vi "WPI_CameraUpdate Settings.vi"(8 "Name":string, 9 "Table":string, 11 "CameraDevRef":T1) -> ()   [LabVIEW 2017]
uses:
  <vilib>/Rock Robotics/WPI/Camera/WPI_CameraDevRef.ctl
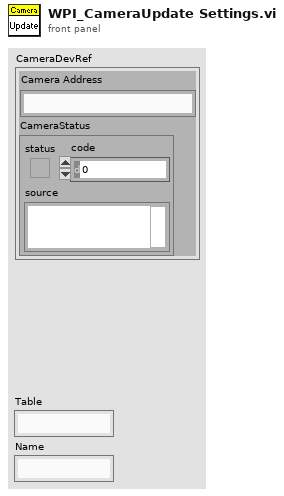
[diagram p1: front panel]
types:
  T1 = typedef "WPI_CameraDevRef.ctl" = cluster{"Camera Address":string, "CameraStatus":errorcluster}
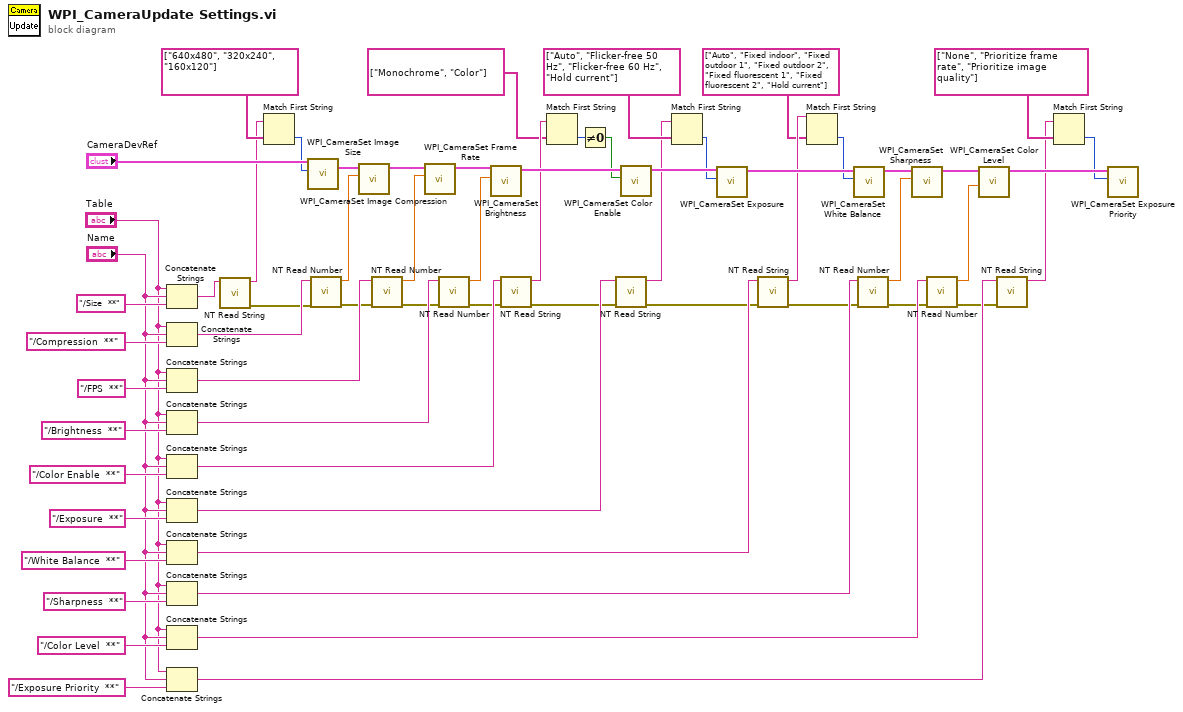
[diagram p0: block diagram]
diagram:
  n1 = Concatenate Strings("Table", "Name", "/Size  **") -> (w40:string)
  n2 = Concatenate Strings("Table", "Name", "/Compression  **") -> (w39:string)
  n3 = Concatenate Strings("Table", "Name", "/FPS  **") -> (w38:string)
  n4 = Concatenate Strings("Table", "Name", "/Brightness  **") -> (w37:string)
  n5 = Concatenate Strings("Table", "Name", "/Color Enable  **") -> (w14:string)
  n6 = Concatenate Strings("Table", "Name", "/Exposure  **") -> (w36:string)
  n7 = Concatenate Strings("Table", "Name", "/White Balance  **") -> (w35:string)
  n8 = Concatenate Strings("Table", "Name", "/Sharpness  **") -> (w34:string)
  n9 = Concatenate Strings("Table", "Name", "/Color Level  **") -> (w33:string)
  n10 = Concatenate Strings("Table", "Name", "/Exposure Priority  **") -> (w32:string)
  n11 = call <vilib>:"NT Read String.vi"("Name"=w40) -> ("error out"=w9:errorcluster, "String"=w19:string)  [unwired: 9 in]
  n12 = Match First String(2:string[] ["640x480", "320x240", "160x120"], 3:w19) -> (0:w18:i32)  [unwired: 1 out]
  n13 = call <vilib>:"WPI_CameraSet Image Size.vi"("Image Size"=w18, "CameraDevRef"="CameraDevRef") -> ("CameraDevRef Out"=w47:T1)  [unwired: 8 in, 1 out]
  n14 = call <vilib>:"NT Read Number.vi"("error in"=w9, "Name"=w39) -> ("error out"=w8:errorcluster, "Numeric"=w31:dbl)  [unwired: 8 in]
  n15 = call <vilib>:"WPI_CameraSet Image Compression.vi"("Compression"=w31, "CameraDevRef"=w47) -> ("CameraDevRef Out"=w48:T1)  [unwired: 8 in, 1 out]
  n16 = call <vilib>:"NT Read Number.vi"("error in"=w8, "Name"=w38) -> ("error out"=w7:errorcluster, "Numeric"=w30:dbl)  [unwired: 8 in]
  n17 = call <vilib>:"WPI_CameraSet Frame Rate.vi"("Frame Rate (fps)"=w30, "CameraDevRef"=w48) -> ("CameraDevRef Out"=w49:T1)  [unwired: 8 in, 1 out]
  n18 = call <vilib>:"NT Read Number.vi"("error in"=w7, "Name"=w37) -> ("error out"=w6:errorcluster, "Numeric"=w29:dbl)  [unwired: 8 in]
  n19 = call <vilib>:"WPI_CameraSet Brightness.vi"("Brightness"=w29, "CameraDevRef"=w49) -> ("CameraDevRef Out"=w46:T1)  [unwired: 8 in, 1 out]
  n20 = call <vilib>:"NT Read String.vi"("error in"=w6, "Name"=w14) -> ("error out"=w5:errorcluster, "String"=w13:string)  [unwired: 8 in]
  n21 = Match First String(2:string[] ["Monochrome", "Color"], 3:w13) -> (0:w10:i32)  [unwired: 1 out]
  n22 = Not Equal To 0?(x=w10) -> (x != 0?=w11:bool)
  n23 = call <vilib>:"NT Read String.vi"("error in"=w5, "Name"=w36) -> ("error out"=w4:errorcluster, "String"=w16:string)  [unwired: 8 in]
  n24 = call <vilib>:"WPI_CameraSet Color Enable.vi"("Color Enabled"=w11, "CameraDevRef"=w46) -> ("CameraDevRef Out"=w45:T1)  [unwired: 8 in, 1 out]
  n25 = Match First String(2:string[] ["Auto", "Flicker-free 50 Hz", "Flicker-free 60 Hz", "Hold current"], 3:w16) -> (0:w15:i32)  [unwired: 1 out]
  n26 = call <vilib>:"WPI_CameraSet Exposure.vi"("Exposure"=w15, "CameraDevRef"=w45) -> ("CameraDevRef Out"=w44:T1)  [unwired: 8 in, 1 out]
  n27 = call <vilib>:"NT Read String.vi"("error in"=w4, "Name"=w35) -> ("error out"=w3:errorcluster, "String"=w23:string)  [unwired: 8 in]
  n28 = Match First String(2:string[] ["Auto", "Fixed indoor", "Fixed outdoor 1", "Fixed outdoor 2", "Fixed fluorescent 1", "Fixed fluorescent 2", "Hold current"], 3:w23) -> (0:w21:i32)  [unwired: 1 out]
  n29 = call <vilib>:"WPI_CameraSet White Balance.vi"("White Balance"=w21, "CameraDevRef"=w44) -> ("CameraDevRef Out"=w43:T1)  [unwired: 8 in, 1 out]
  n30 = call <vilib>:"NT Read Number.vi"("error in"=w3, "Name"=w34) -> ("error out"=w2:errorcluster, "Numeric"=w28:dbl)  [unwired: 8 in]
  n31 = call <vilib>:"WPI_CameraSet Sharpness.vi"("Sharpness"=w28, "CameraDevRef"=w43) -> ("CameraDevRef Out"=w42:T1)  [unwired: 8 in, 1 out]
  n32 = call <vilib>:"NT Read Number.vi"("error in"=w2, "Name"=w33) -> ("error out"=w1:errorcluster, "Numeric"=w27:dbl)  [unwired: 8 in]
  n33 = call <vilib>:"WPI_CameraSet Color Level.vi"("Color Level"=w27, "CameraDevRef"=w42) -> ("CameraDevRef Out"=w41:T1)  [unwired: 8 in, 1 out]
  n34 = call <vilib>:"NT Read String.vi"("error in"=w1, "Name"=w32) -> ("String"=w25:string)  [unwired: 8 in, 1 out]
  n35 = Match First String(2:string[] ["None", "Prioritize frame rate", "Prioritize image quality"], 3:w25) -> (0:w24:i32)  [unwired: 1 out]
  n36 = call <vilib>:"WPI_CameraSet Exposure Priority.vi"("Exposure Priority"=w24, "CameraDevRef"=w41) -> ()  [unwired: 8 in, 2 out]
